vi "Subvi Insert Suffix in Filename.vi"(1 "Exposure":dbl, 2 "OnlyROI":bool, 3 "Suffix":string, 4 "InFileName":string) -> (0 "OutFileName":string)   [LabVIEW 2012]
uses:
  ProSCI Global.vi
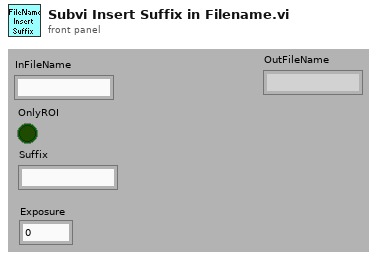
[diagram p1: front panel]
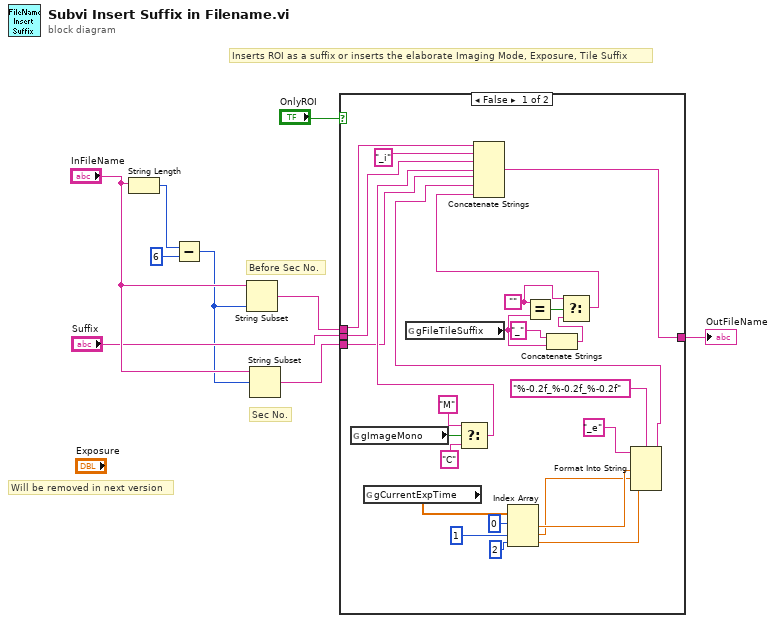
[diagram p0: block diagram]
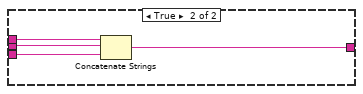
[diagram p2: hidden frame]
diagram:
  # "Will be removed in next version"
  # "Before Sec No."
  # "Sec No."
  # "Inserts ROI as a suffix or inserts the elaborate Imaging Mode, Exposure, Tile Suffix"
  n1 = String Length(string="InFileName") -> (length=w6:i32)
  n2 = Subtract(x=w6, y=6) -> (x-y=w4:i32)
  n3 = String Subset(string="InFileName", length (rest)=w4) -> (substring=w3:string)  [unwired: 1 out]
  n4 = String Subset(string="InFileName", offset (0)=w4) -> (substring=w2:string)  [unwired: 1 out]
  n5 = case shown="False" "OnlyROI" {
    tunnel: "Suffix" -> [w32 w38]
    tunnel: [w17 w37] -> w7
    tunnel: w3 -> [w34 w36]
    tunnel: w2 -> [w27 w35]
    frame False {
      w21 = ""
      n6 = global read "ProSCI Global.vi" "gImageMono"() -> (w31:bool)
      n7 = global read "ProSCI Global.vi" "gCurrentExpTime"() -> (w16:dbl[])
      n8 = global read "ProSCI Global.vi" "gFileTileSuffix"() -> (w23:string)
      n9 = Select(t="M" ("initial string"), s=w31, f="C" ("initial string")) -> (s? t:f=w28:string)
      n10 = Index Array(array=w16, index #1=0, index #2=1, index #3=2) -> (element #1=w12:dbl, element #2=w11:dbl, element #3=w10:dbl)
      n11 = Equal?(x=w21, y=w23) -> (x = y?=w19:bool)
      n12 = Concatenate Strings("_" ("format string"), w23) -> (w20:string)
      n13 = Select(t=w21, s=w19, f=w20) -> (s? t:f=w18:string)
      n14 = Format Into String(format string="%-0.2f_%-0.2f_%-0.2f", initial string="_e", w12, w11, w10) -> (resulting string=w24:string)  [unwired: 1 in, 1 out]
      n15 = Concatenate Strings(w34, "_i" ("format string"), w32, w28, w27, w24, w18) -> (w17:string)
    }
    frame True {
      n16 = Concatenate Strings(w36, w38, w35) -> (w37:string)
    }
  }
  "OutFileName" <- w7
